vi "Find all New Corners.vi"(3 "Points":cluster{"Col":i8, "Row":i8}[](array[cluster]), 4 "# safety grids":i32, 5 "Updated Map":i8[][](array[numeric])) -> (1 "Corners":cluster{"Col":i8, "Row":i8}[](array[cluster]))   [LabVIEW 2009]
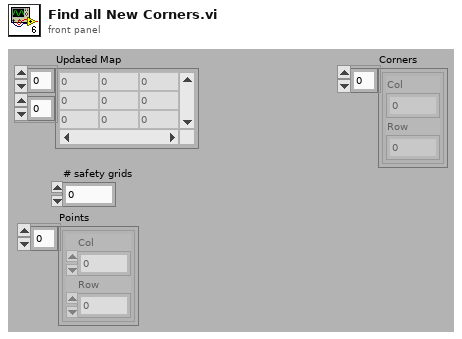
[diagram p1: front panel]
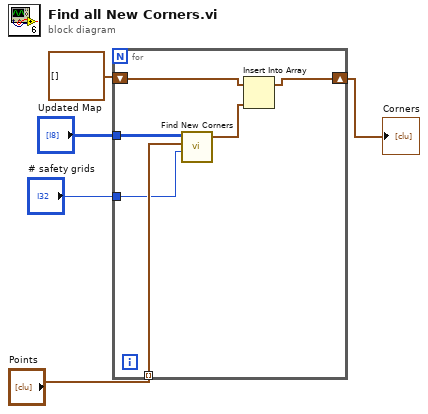
[diagram p0: block diagram]
diagram:
  n1 = for {
    tunnel: "Updated Map" -> [w11]
    tunnel: "Points" -> [w10] mode=indexing
    shift-right: [w8] -> w3
    shift-left: cluster{"Col":i8, "Row":i8}[] [] -> [w7]
    tunnel: "# safety grids" -> [w6]
    n2 = call "Find New Corners.vi"("Updated Map"=w11, "Point"=w10, "# safety grids"=w6) -> ("Corners"=w9:cluster{"Col":dbl, "Row":dbl}[])  [unwired: 3 in]
    n3 = Insert Into Array(array=w7, new element=w9) -> (w8:cluster{"Col":i8, "Row":i8}[])  [unwired: 1 in]
  }
  "Corners" <- w3
